vi "Ctr sys net adapter port auto detect.vi"(11 "Sys Config to save in":T1={"XY Stage"={"COM port"="", "XY stage available"=FALSE}, "DAQ FPGA"={"Ref"=refnum, "Target"="RIO0", "Clock Freq (MHz) "=200.0, "input card type"=enum."AC Card", "Samples Wait after Trigger"=5080, "AOD fill"=4900, "StartupDelay"=0, "Slip Cycle (clock cycles)"=600000, "Add Cycle"=TRUE}, "Control system"={"Ethernet opened"=FALSE, "Ethernet Port"=3, "Ctrl FPGA available"=FALSE, "Ctrl FPGA Clock (MHz)"=240.0, "Ctrl system MAC address"="", "Control system.Network adapter name"="", "AOD 1 Amplitude"=0, "AOD 2 Amplitude"=0, "AOD 3 Amplitude"=0, "AOD 4 Amplitude"=0, "Data Time Interval (ns)"=0.0, "T0 (ns)"=0.0, "Ta (ns)"=0.0}, "Encoder"={"IP address"="224.0.1.103", "Port"=7000, "Encoder available"=FALSE, "Wheel radius (cm)"=16.0}, "DAQmx Chan"={"Pockels AO"="", "Hard shutter AO"="", "PMT AOs"="", "Power meter AI"=""}, "Computer MAC address"="", "Cam VidRec"={"DO flag-Video record"="", "DO flag-Trial start"="", "VidRec available"=FALSE}, "Externalise Triggers"=FALSE, "Laser wavelength (nm)"=920.0} {"Laser wavelength (nm)" min=800.0 max=1080.0 step=1.0; "Encoder"."Wheel radius (cm)" format="%#_13g"; "Control system"."Ctrl FPGA Clock (MHz)" min=80.0 max=500.0 step=1.0; "Control system"."Data Time Interval (ns)" min=0.0 max=2048.0 step=1.0; "Control system"."Ta (ns)" min=0.0 max=2048.0 step=1.0; "Control system"."T0 (ns)" min=0.0 max=2048.0 step=1.0; "Control system"."AOD 4 Amplitude" min=0 max=2048 step=1; "Control system"."AOD 3 Amplitude" min=0 max=2048 step=1; "Control system"."AOD 2 Amplitude" min=0 max=2048 step=1; "Control system"."AOD 1 Amplitude" min=0 max=2048 step=1}) -> (0 "error out":errorcluster, 3 "Sys Config to save out":T1={"XY Stage"={"COM port"="", "XY stage available"=FALSE}, "DAQ FPGA"={"Ref"=refnum, "Target"="RIO0", "Clock Freq (MHz) "=200.0, "input card type"=enum."AC Card", "Samples Wait after Trigger"=5080, "AOD fill"=4900, "StartupDelay"=0, "Slip Cycle (clock cycles)"=600000, "Add Cycle"=TRUE}, "Control system"={"Ethernet opened"=FALSE, "Ethernet Port"=3, "Ctrl FPGA available"=FALSE, "Ctrl FPGA Clock (MHz)"=240.0, "Ctrl system MAC address"="", "Control system.Network adapter name"="", "AOD 1 Amplitude"=0, "AOD 2 Amplitude"=0, "AOD 3 Amplitude"=0, "AOD 4 Amplitude"=0, "Data Time Interval (ns)"=0.0, "T0 (ns)"=0.0, "Ta (ns)"=0.0}, "Encoder"={"IP address"="224.0.1.103", "Port"=7000, "Encoder available"=FALSE, "Wheel radius (cm)"=16.0}, "DAQmx Chan"={"Pockels AO"="", "Hard shutter AO"="", "PMT AOs"="", "Power meter AI"=""}, "Computer MAC address"="", "Cam VidRec"={"DO flag-Video record"="", "DO flag-Trial start"="", "VidRec available"=FALSE}, "Externalise Triggers"=FALSE, "Laser wavelength (nm)"=920.0} {"Laser wavelength (nm)" min=800.0 max=1080.0 step=1.0; "Encoder"."Wheel radius (cm)" format="%#_13g"; "Control system"."Ctrl FPGA Clock (MHz)" min=80.0 max=500.0 step=1.0; "Control system"."Data Time Interval (ns)" min=0.0 max=2048.0 step=1.0; "Control system"."Ta (ns)" min=0.0 max=2048.0 step=1.0; "Control system"."T0 (ns)" min=0.0 max=2048.0 step=1.0; "Control system"."AOD 4 Amplitude" min=0 max=2048 step=1; "Control system"."AOD 3 Amplitude" min=0 max=2048 step=1; "Control system"."AOD 2 Amplitude" min=0 max=2048 step=1; "Control system"."AOD 1 Amplitude" min=0 max=2048 step=1})   [LabVIEW 2013]
uses:
  Typedefs/Sys Configuration.ctl
  Typedefs/XY Stage config cluster.ctl
  Typedefs/DAQ FPGA config cluster.ctl
  RIG-SPECIFIC FILES/FPGA Refs/FPGA Ref.ctl
  <vilib>/userdefined/High Color/nirio_resource_hc.ctl
  Typedefs/FPGA input type AC-DC.ctl
  Typedefs/CTRL system config cluster.ctl
  Typedefs/Encoder config cluster.ctl
  Typedefs/DAQmx physical channels cluster.ctl
  Typedefs/Cam VidRec HW config setup cluster.ctl
  Global Variables/General Globals.vi
panel:
  out "Control system's network adapter name":string="82574L"
  out "Ethernet opened":bool
  out "# of enabled ports":i32
  out "Port Number":u32
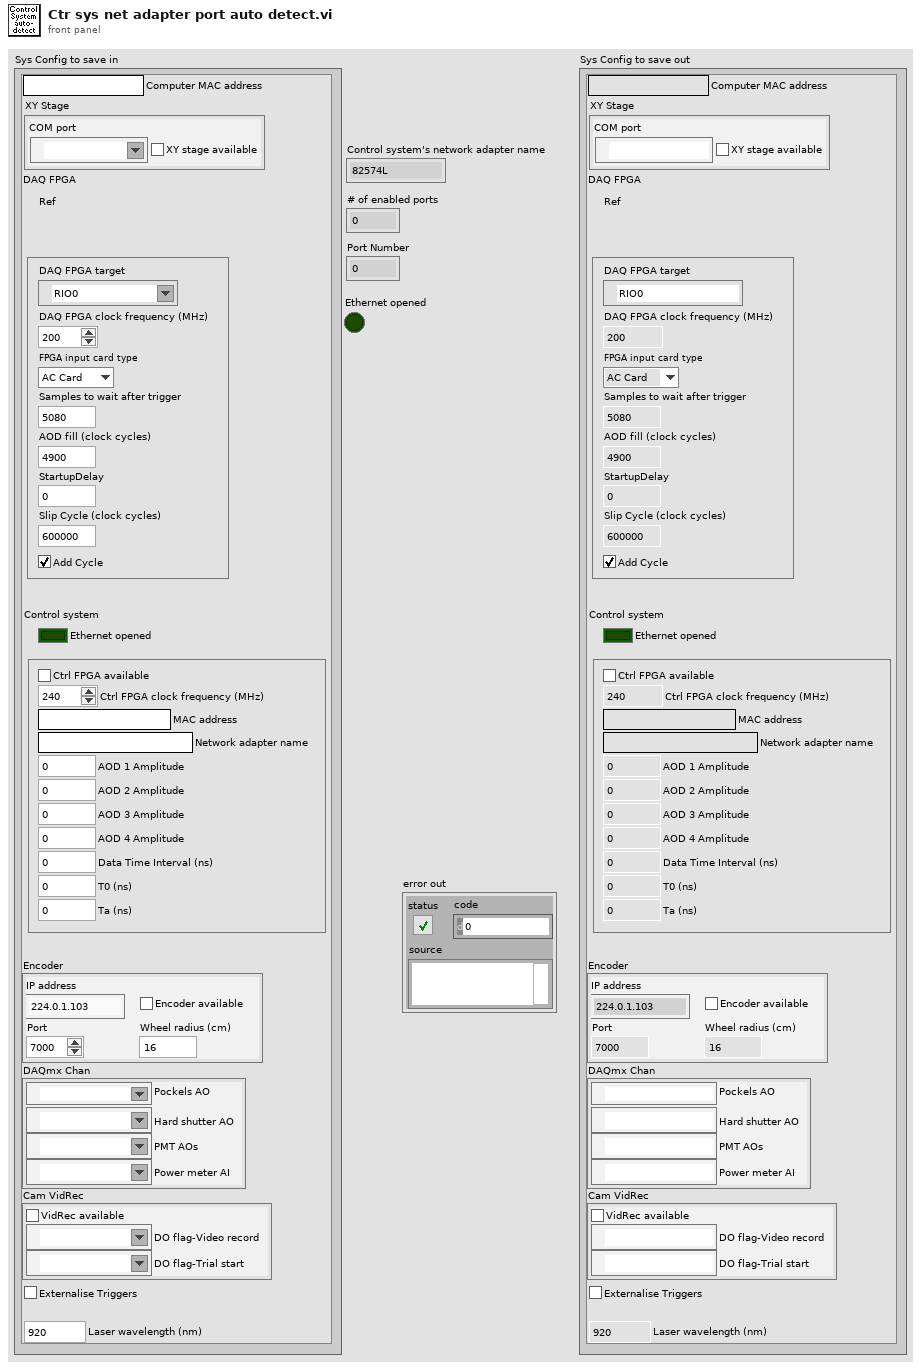
[diagram p1: front panel]
types:
  T1 = typedef "Sys Configuration.ctl" = cluster{"XY Stage":T2, "DAQ FPGA":T3, "Control system":T7, "Encoder":T8, "DAQmx Chan":T9, "Computer MAC address":string, "Cam VidRec":T10, "Externalise Triggers":bool, "Laser wavelength (nm)":dbl}
  T2 = typedef "XY Stage config cluster.ctl" = cluster{"COM port":refnum<visa-resource-name>, "XY stage available":bool}
  T3 = typedef "DAQ FPGA config cluster.ctl" = cluster{"Ref":T4, "Target":T5, "Clock Freq (MHz) ":dbl, "input card type":T6, "Samples Wait after Trigger":u16, "AOD fill":u16, "StartupDelay":i32, "Slip Cycle (clock cycles)":u32, "Add Cycle":bool}
  T4 = typedef "FPGA Ref.ctl" = refnum<k20>
  T5 = typedef "nirio_resource_hc.ctl" = tag
  T6 = typedef "FPGA input type AC-DC.ctl" = enum16{"AC Card", "DC Card"}
  T7 = typedef "CTRL system config cluster.ctl" = cluster{"Ethernet opened":bool, "Ethernet Port":u32, "Ctrl FPGA available":bool, "Ctrl FPGA Clock (MHz)":dbl, "Ctrl system MAC address":string, "Control system.Network adapter name":string, "AOD 1 Amplitude":i16, "AOD 2 Amplitude":i16, "AOD 3 Amplitude":i16, "AOD 4 Amplitude":i16, "Data Time Interval (ns)":dbl, "T0 (ns)":dbl, "Ta (ns)":dbl}
  T8 = typedef "Encoder config cluster.ctl" = cluster{"IP address":string, "Port":u16, "Encoder available":bool, "Wheel radius (cm)":dbl}
  T9 = typedef "DAQmx physical channels cluster.ctl" = cluster{"Pockels AO":tag, "Hard shutter AO":tag, "PMT AOs":tag, "Power meter AI":tag}
  T10 = typedef "Cam VidRec HW config setup cluster.ctl" = cluster{"DO flag-Video record":tag, "DO flag-Trial start":tag, "VidRec available":bool}
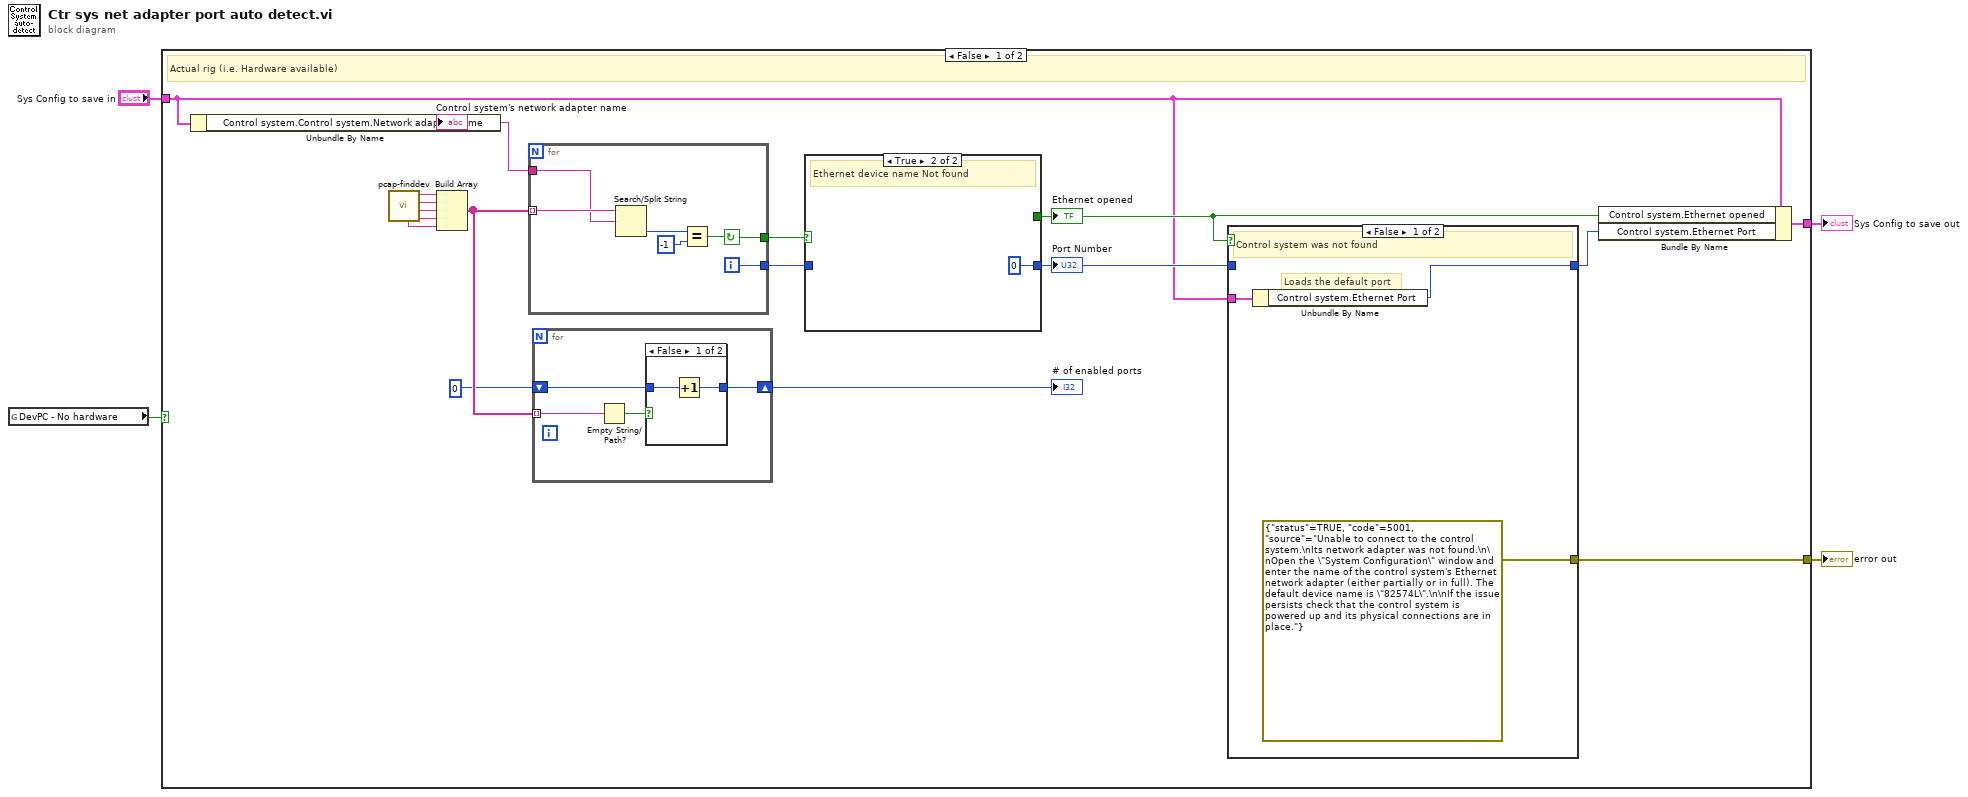
[diagram p0: block diagram]
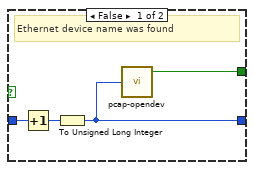
[diagram p4: hidden frame]
diagram:
  n1 = global read "General Globals.vi" "DevPC - No hardware"() -> (w1:bool)
  n2 = case shown="False" w1 {
    tunnel: [w11 w44] -> w4
    tunnel: "Sys Config to save in" -> [w7 w44]
    tunnel: [w6 _] -> w2
    frame False {
      # "Actual rig (i.e. Hardware available)"
      n3 = Unbundle By Name(w7) -> ("Control system.Control system.Network adapter name"=w5:string)
      "Control system's network adapter name" <- w5
      n4 = call "pcap-finddev.vi"() -> ("String 4"=w18:string, "String 3"=w19:string, "String 2"=w20:string, "String"=w21:string, "String 5"=w17:string)  [unwired: 1 in]
      n5 = Build Array(w21, w20, w19, w18, w17) -> (w14:string[])
      n6 = for {
        tunnel: w14 -> [w39] mode=indexing
        tunnel: [w41] -> w16
        tunnel: [w40] -> w15
        tunnel: w5 -> [w38]
        i -> [w40]
        stop <- w41 continue-if-true
        n7 = Search/Split String(string=w39, search string/char (-)=w38) -> (offset of match=w43:i32)  [unwired: 1 in, 2 out]
        n8 = Equal?(x=w43, y=-1) -> (x = y?=w41:bool)
      }
      n9 = for {
        shift-right: [w28] -> w12
        shift-left: 0 -> [w27]
        tunnel: w14 -> [w26] mode=indexing
        n10 = Empty String/Path?(string/path=w26) -> (empty?=w29:bool)
        n11 = case shown="False" w29 {
          tunnel: [w31 w32] -> w28
          tunnel: w27 -> [w30 w32]
          frame False {
            n12 = Increment(x=w30) -> (x+1=w31:i32)
          }
          frame True {
          }
        }
      }
      "# of enabled ports" <- w12
      n13 = case shown="True" w16 {
        tunnel: w15 -> [w36 _]
        tunnel: [w33 u32 0] -> w9
        tunnel: [w35 _] -> w10
        frame False {
          # "Ethernet device name was found"
          n14 = Increment(x=w36) -> (x+1=w34:i32)
          n15 = To Unsigned Long Integer(number=w34) -> (unsigned 32bit integer=w33:u32)
          n16 = call "pcap-opendev.vi"("Select Device"=w33) -> ("Opened"=w35:bool)  [unwired: 2 out]
        }
        frame True {
          # "Ethernet device name Not found"
        }
      }
      "Port Number" <- w9
      "Ethernet opened" <- w10
      n17 = case shown="False" w10 {
        tunnel: [w23 w25] -> w8
        tunnel: w9 -> [_ w25]
        tunnel: w7 -> [w24 _]
        tunnel: [errorcluster {"status"=TRUE, "code"=5001, "source"="Unable to connect to the control system.\nIts network adapter was not found.\n\nOpen the \"System Configuration\" window and enter the name of the control system's Ethernet network adapter (either partially or in full). The default device name is \"82574L\".\n\nIf the issue persists check that the control system is powered up and its physical connections are in place."} ("error in (no error)") _] -> w6
        frame False {
          # "Loads the default port"
          # "Control system was not found"
          n18 = Unbundle By Name(w24) -> ("Control system.Ethernet Port"=w23:u32)
        }
        frame True {
          # "Control system was found"
        }
      }
      n19 = Bundle By Name(cluster=w7, "Control system.Ethernet opened"=w10, "Control system.Ethernet Port"=w8) -> (w11:T1)
    }
    frame True {
      # "Development Computer (i.e. No hardware available)"
    }
  }
  "Sys Config to save out" <- w4
  "error out" <- w2
